vi "RT_Transmission.vi"() -> ()   [LabVIEW 2016]
uses:
  <vilib>/Instr/_visa.llb/VISA Configure Serial Port (Instr).vi
  <vilib>/FPGAPlugInAG/cRIO-9067/niLvFpga_Open_cRIO-9067.vi
  <vilib>/Utility/error.llb/Error Cluster From Error Code.vi
  <vilib>/rvi/errors/niLvFpgaAdjustHostInterfaceError.vi
  <vilib>/functionblocks/Control/PID/PID.vi
  <vilib>/rvi/interface/nirviOpenFPGA/nirviOpenFPGA.xnode
  FPGA Bitfiles/MayUpgrade_FPGA-Trans_Transmission-FPG_MZXtHOBdRVI.lvbitx
  FPGA_Transmission.vi
  <vilib>/rvi/interface/nirviReadWriteControl/nirviReadWriteControl.xnode
  <vilib>/functionblocks/FB Core/FB Core.xnode
  <vilib>/functionblocks/NI_FunctionBlock Libraries.lvlib
  NiFpgaLv.dll
  <vilib>/rvi/errors/niLvFpgaMergeErrorWithErrorCode.vi
panel:
  in  "Tab Control":enum32{"control", "Junk"}(tab)
  out "Steerer X+":dbl
  out "Steerer X-":dbl
  out "Steerer Y+":dbl
  out "Steerer Y-":dbl
  out "ExB +":dbl
  out "ExB -":dbl
  out "X+ V":fxp<+/-,26,5> format="%.23g"
  out "X+ I":fxp<+/-,26,5> format="%_4g"
  out "X- V":fxp<+/-,26,5> format="%_4g"
  out "X-I":fxp<+/-,26,5> format="%_4g"
  out "Y+ V":fxp<+/-,26,5> format="%_4g"
  out "Y+I":fxp<+/-,26,5> format="%_4g"
  out "Y-V":fxp<+/-,26,5> format="%_4g"
  out "Y-I":fxp<+/-,26,5> format="%_4g"
  out "ExB + V":fxp<+/-,26,5> format="%_4g"
  out "ExB +I":fxp<+/-,26,5> format="%_4g"
  out "ExB -V":fxp<+/-,26,5> format="%_4g"
  out "ExB-I":fxp<+/-,26,5> format="%_4g"
  out "concatenated string":string
  out "Ion gauge switch object cluser 2":T1
  out "Ion gauge anal waist Cluster 1":T1
  out "EXB":dbl
  in  "derivative time (Td, min)":dbl=0.05
  in  "integral time (Ti, min)":dbl=0.01
  in  "proportional gain (Kc)":dbl=25.0
  out "concatenated string 2":string
  out "anal field read":dbl
  out "unsigned byte array":u8[](array[numeric])
  out "Analyze read":u8[](array[numeric])
  out "analyze magnet set field":dbl
  out "element":dbl
  in  "diverter":bool
  out "diverter":bool
  out "ExB loop error":errorcluster
  out "Analog control error":errorcluster
  out "FPGA error":errorcluster
  in  "Ion gauge cluster control":T1
  out "Convectron 3":u8[](array[numeric])
  out "Ion gauge 4":u8[](array[numeric])
  out "Convectron 4":u8[](array[numeric])
  out "Ion gauge 5":u8[](array[numeric])
  out "Convectron 2":u8[](array[numeric])
  out "Ion gauge 2":u8[](array[numeric])
  out "Convectron 1":u8[](array[numeric])
  out "Ion gauge 1":u8[](array[numeric])
  out "Vac Cluster Error":errorcluster
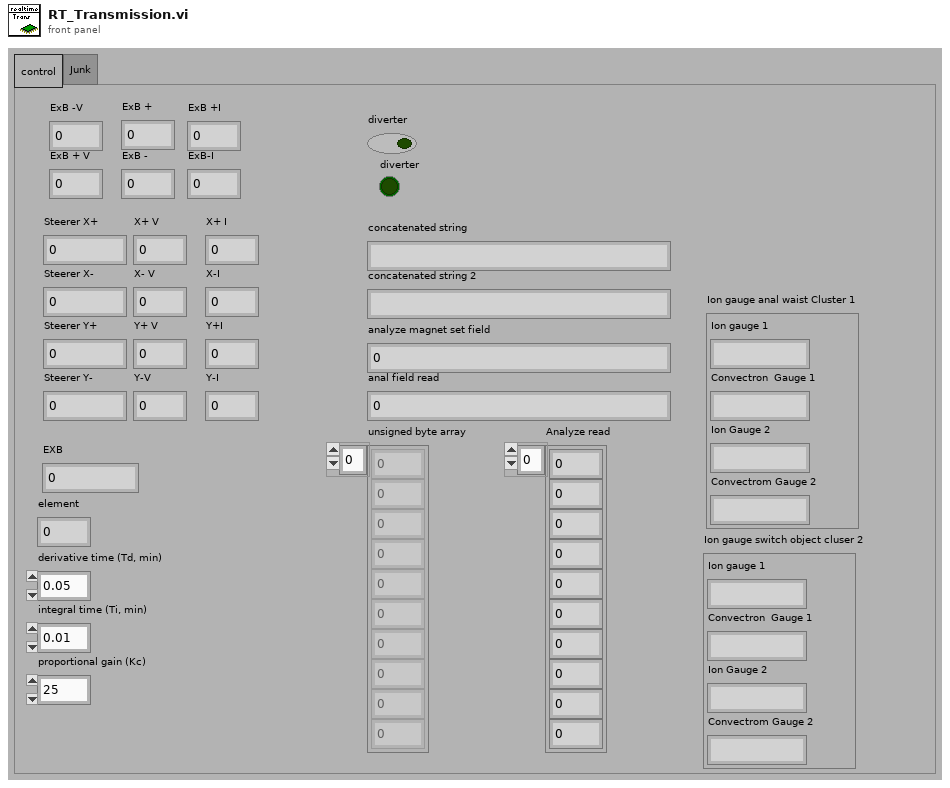
[diagram p1: front panel]
types:
  T1 = cluster{"Ion gauge 1":string, "Convectron  Gauge 1 ":string, "Ion Gauge 2":string, "Convectrom Gauge 2":string}
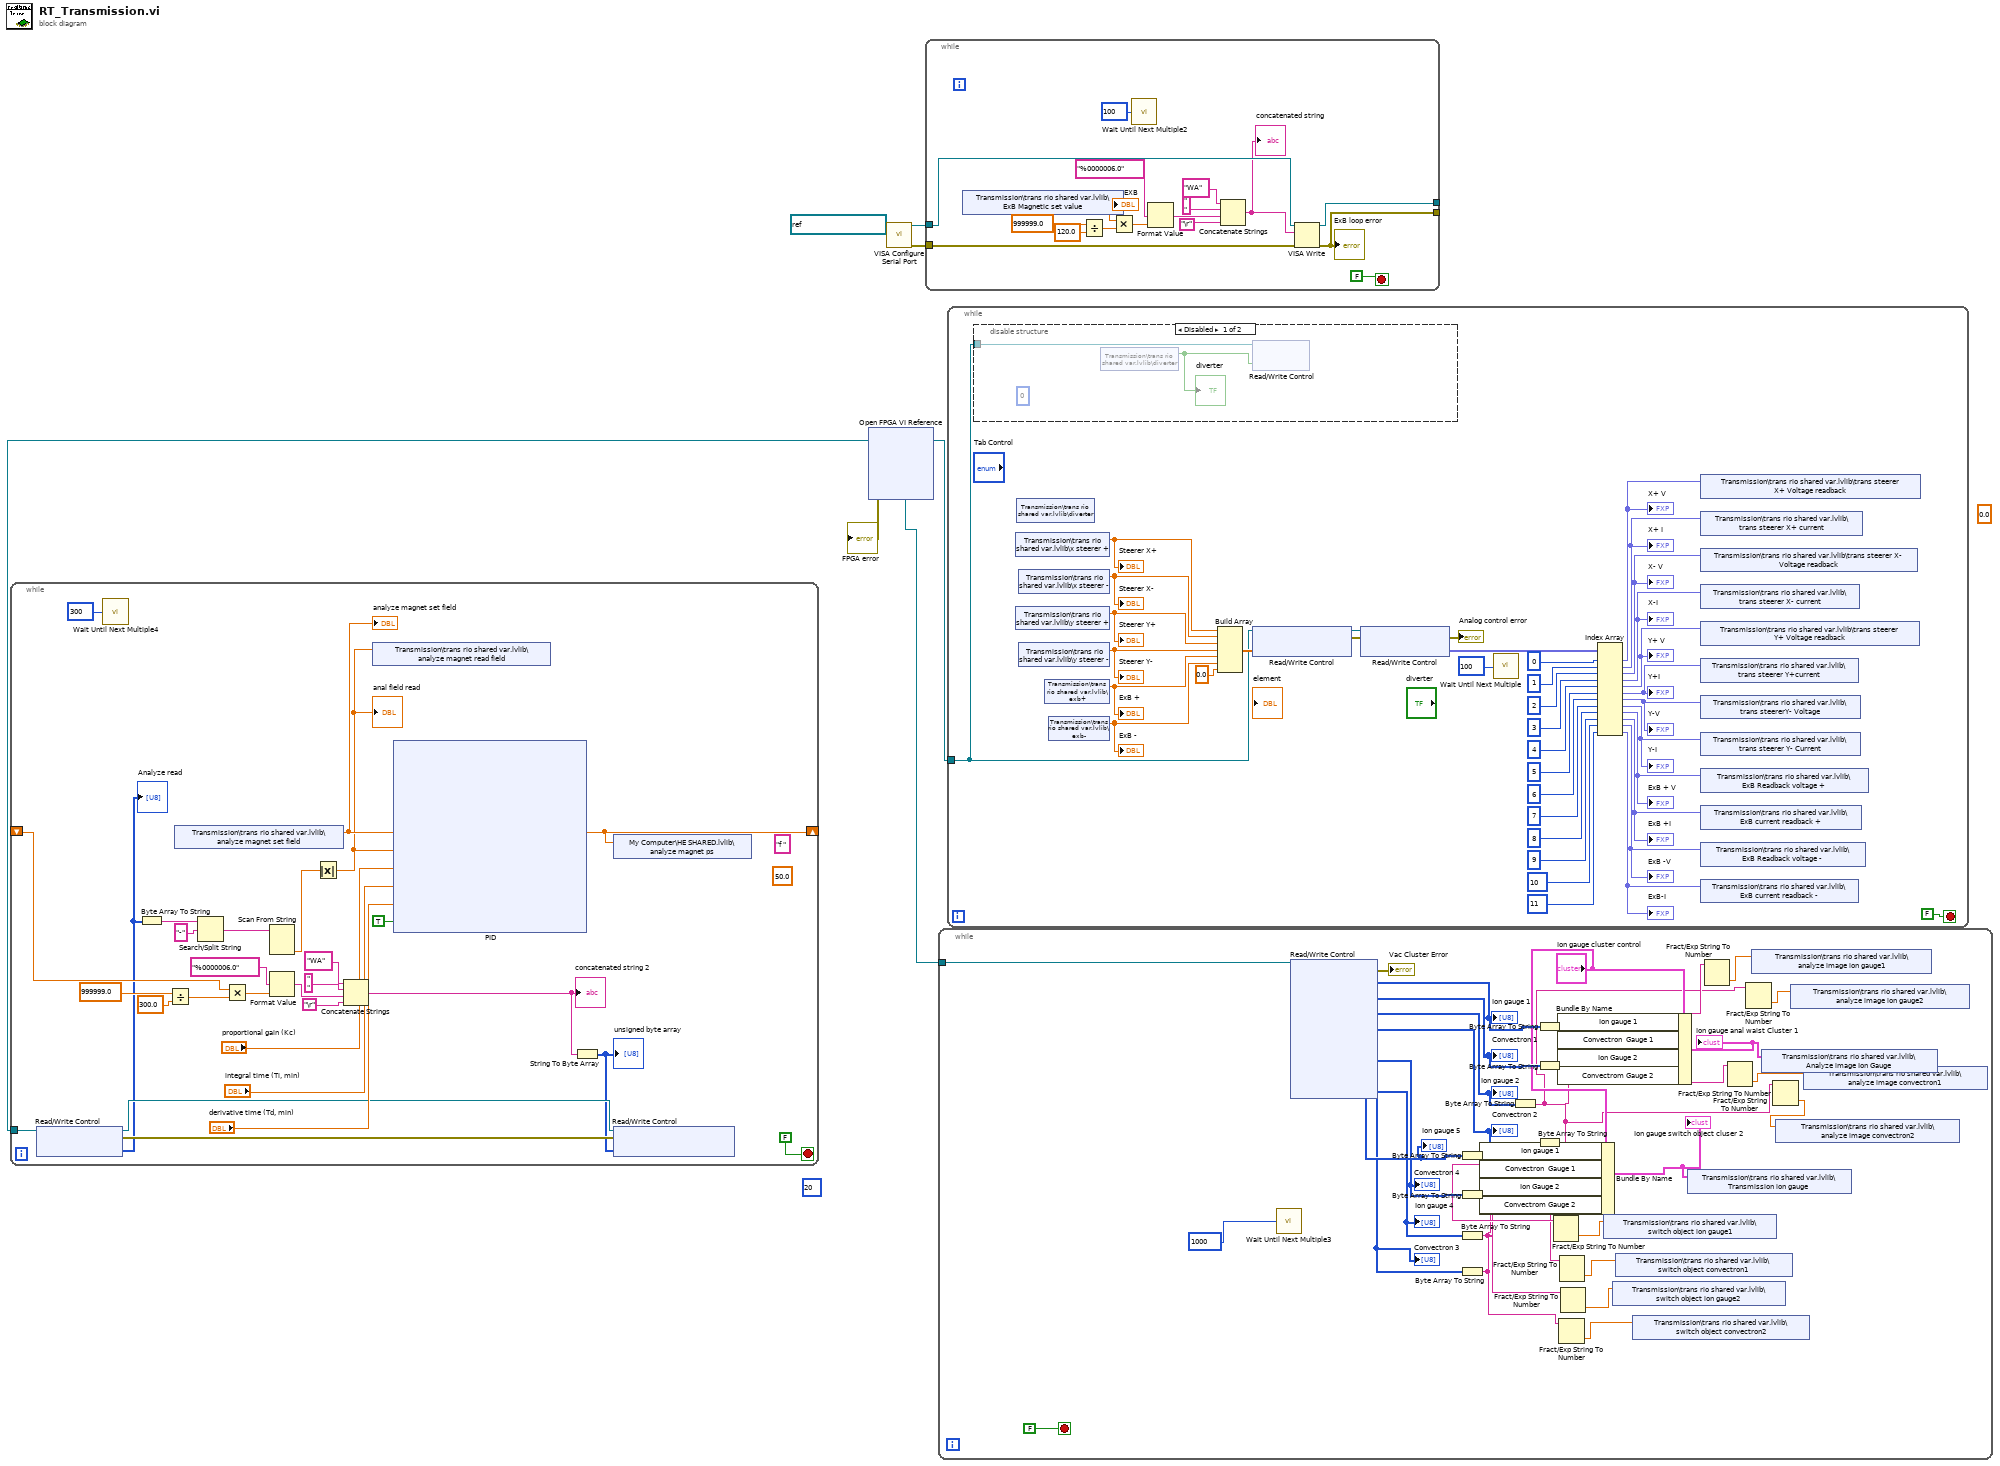
[diagram p0: block diagram]
diagram:
  (unwired) 20 ("dimension size")
  (unwired) 0.0 ("output")
  n1 = xnode "Open FPGA VI Reference"() -> ("FPGA VI Reference Out"=w1:refnum<k20>, "error out"=→"FPGA error":errorcluster)  [unwired: 2 in]
  n2 = while {
    shift-right: [w20] -> _
    shift-left: _ -> [w9]
    tunnel: w1 -> [w14]
    stop <- FALSE stop-if-true
    (unwired) 50.0 ("x")
    (unwired) "f " ("regular expression")
    n3 = xnode "Read/Write Control"("FPGA VI Reference In"=w14) -> ("FPGA VI Reference Out"=w13:refnum<k20>, "error out"=w12:errorcluster, "Analyze read"=w8:u8[])  [unwired: 1 in]
    "Analyze read" <- w8
    n4 = call "Wait Until Next Multiple4"("Count(mSec)"=u32 300 ("millisecond multiple")) -> ()  [unwired: 1 out]
    n5 = Byte Array To String(unsigned byte array=w8) -> (string=w22:string)
    n6 = Divide(x=999999.0, y=300.0) -> (x/y=w27:dbl)
    n7 = shared-variable "Transmission\\trans rio shared var.lvlib\\analyze magnet set field"() -> (w7:dbl)  [unwired: 1 in, 1 out]
    "analyze magnet set field" <- w7
    n8 = Search/Split String(string=w22, search string/char (-)="-") -> (match + rest of string=w10:string)  [unwired: 3 out]
    n9 = Multiply(x=w9, y=w27) -> (x*y=w29:dbl)
    n10 = Scan From String(input string=w10) -> (output 1=w21:dbl)  [unwired: 3 in, 4 out]
    n11 = Format Value(format string="%0000006.0", value (0)=w29) -> (output string=w32:string)  [unwired: 1 out]
    n12 = Absolute Value(x=w21) -> (abs(x)=w6:dbl)
    "anal field read" <- w6
    n13 = Concatenate Strings("WA", " ", w32, "\r") -> (w33:string)
    "concatenated string 2" <- w33
    n14 = shared-variable "Transmission\\trans rio shared var.lvlib\\analyze magnet read field"(w6) -> ()  [unwired: 1 in, 1 out]
    n15 = xnode "PID"("setpoint"=w7, "process variable"=w6, "proportional gain (Kc)"="proportional gain (Kc)", "integral time (Ti, min)"="integral time (Ti, min)", "derivative time (Td, min)"="derivative time (Td, min)", "auto? (T)"=TRUE) -> ("output"=w20:dbl)  [unwired: 1 in, 1 out]
    n16 = String To Byte Array(string=w33) -> (unsigned byte array=w11:u8[])
    "unsigned byte array" <- w11
    n17 = shared-variable "My Computer\\HE SHARED.lvlib\\analyze magnet ps"(w20) -> ()  [unwired: 1 in, 1 out]
    n18 = xnode "Read/Write Control"("FPGA VI Reference In"=w13, "error in"=w12, "analyze ps set array"=w11) -> ()  [unwired: 2 out]
  }
  n19 = call-poly "VISA Configure Serial Port"("VISA resource name"=refnum<visa-resource-name> "ASRL1::INSTR") -> ("VISA resource name out"=w5:refnum<visa-resource-name>, "error out"=w4:errorcluster)  [unwired: 5 in, 8 out]
  n20 = while {
    tunnel: w4 -> [w107]
    tunnel: w5 -> [w106]
    tunnel: [w104] -> _
    tunnel: [w103] -> _
    stop <- FALSE stop-if-true
    n21 = shared-variable "Transmission\\trans rio shared var.lvlib\\ExB Magnetic set value"() -> (w102:dbl)  [unwired: 1 in, 1 out]
    "EXB" <- w102
    n22 = Divide(x=999999.0, y=120.0) -> (x/y=w115:dbl)
    n23 = Multiply(x=w102, y=w115) -> (x*y=w108:dbl)
    n24 = call "Wait Until Next Multiple2"("Count(mSec)"=u32 100) -> ()  [unwired: 1 out]
    n25 = Format Value(format string="%0000006.0", value (0)=w108) -> (output string=w111:string)  [unwired: 1 out]
    n26 = Concatenate Strings("WA", " ", w111, "\r") -> (w105:string)
    "concatenated string" <- w105
    n27 = VISA Write(VISA resource name=w106, write buffer=w105, error in (no error)=w107) -> (VISA resource name out=w104:refnum<visa-resource-name>, error out=w103:errorcluster)  [unwired: 1 out]
    "ExB loop error" <- w103
  }
  n28 = while {
    tunnel: w1 -> [w136]
    stop <- FALSE stop-if-true
    n29 = call "Wait Until Next Multiple3"("Count(mSec)"=u32 1000 ("millisecond multiple")) -> ()  [unwired: 1 out]
    n30 = xnode "Read/Write Control"("FPGA VI Reference In"=w136) -> ("error out"=→"Vac Cluster Error":errorcluster, "Ion gauge 1"=w145:u8[], "Convectron 1"=w146:u8[], "Ion gauge 2"=w147:u8[], "Convectron 2"=w148:u8[], "Ion gauge 3"=w142:u8[], "Convectron 3"=w141:u8[], "Convectron 4"=w139:u8[], "Ion gauge 4"=w140:u8[])  [unwired: 1 in, 1 out]
    "Ion gauge 1" <- w145
    "Convectron 1" <- w146
    "Ion gauge 2" <- w147
    "Convectron 2" <- w148
    "Ion gauge 5" <- w142
    "Convectron 4" <- w141
    "Ion gauge 4" <- w140
    "Convectron 3" <- w139
    n31 = Byte Array To String(unsigned byte array=w142) -> (string=w133:string)
    n32 = Byte Array To String(unsigned byte array=w141) -> (string=w132:string)
    n33 = Byte Array To String(unsigned byte array=w140) -> (string=w131:string)
    n34 = Byte Array To String(unsigned byte array=w139) -> (string=w130:string)
    n35 = Bundle By Name(cluster="Ion gauge cluster control", "Ion gauge 1"=w133, "Convectron  Gauge 1"=w132, "Ion Gauge 2"=w131, "Convectrom Gauge 2"=w130) -> (w135:T1)
    "Ion gauge switch object cluser 2" <- w135
    n36 = Byte Array To String(unsigned byte array=w147) -> (string=w122:string)
    n37 = Byte Array To String(unsigned byte array=w145) -> (string=w125:string)
    n38 = Byte Array To String(unsigned byte array=w146) -> (string=w124:string)
    n39 = Byte Array To String(unsigned byte array=w148) -> (string=w123:string)
    n40 = Fract/Exp String To Number(string=w133) -> (number=w129:dbl)  [unwired: 3 in, 1 out]
    n41 = Bundle By Name(cluster="Ion gauge cluster control", "Ion gauge 1"=w125, "Convectron  Gauge 1"=w124, "Ion Gauge 2"=w122, "Convectrom Gauge 2"=w123) -> (w134:T1)
    "Ion gauge anal waist Cluster 1" <- w134
    n42 = Fract/Exp String To Number(string=w130) -> (number=w126:dbl)  [unwired: 3 in, 1 out]
    n43 = Fract/Exp String To Number(string=w132) -> (number=w128:dbl)  [unwired: 3 in, 1 out]
    n44 = Fract/Exp String To Number(string=w131) -> (number=w127:dbl)  [unwired: 3 in, 1 out]
    n45 = shared-variable "Transmission\\trans rio shared var.lvlib\\switch object ion gauge1"(w129) -> ()  [unwired: 1 in, 1 out]
    n46 = shared-variable "Transmission\\trans rio shared var.lvlib\\switch object ion gauge2"(w127) -> ()  [unwired: 1 in, 1 out]
    n47 = shared-variable "Transmission\\trans rio shared var.lvlib\\switch object convectron1"(w128) -> ()  [unwired: 1 in, 1 out]
    n48 = shared-variable "Transmission\\trans rio shared var.lvlib\\switch object convectron2"(w126) -> ()  [unwired: 1 in, 1 out]
    n49 = shared-variable "Transmission\\trans rio shared var.lvlib\\Transmission ion gauge"(w135) -> ()  [unwired: 1 in, 1 out]
    n50 = Fract/Exp String To Number(string=w125) -> (number=w121:dbl)  [unwired: 3 in, 1 out]
    n51 = Fract/Exp String To Number(string=w124) -> (number=w119:dbl)  [unwired: 3 in, 1 out]
    n52 = Fract/Exp String To Number(string=w122) -> (number=w120:dbl)  [unwired: 3 in, 1 out]
    n53 = shared-variable "Transmission\\trans rio shared var.lvlib\\analyze image ion gauge1"(w121) -> ()  [unwired: 1 in, 1 out]
    n54 = shared-variable "Transmission\\trans rio shared var.lvlib\\Analyze image Ion Gauge"(w134) -> ()  [unwired: 1 in, 1 out]
    n55 = Fract/Exp String To Number(string=w123) -> (number=w118:dbl)  [unwired: 3 in, 1 out]
    n56 = shared-variable "Transmission\\trans rio shared var.lvlib\\analyze image convectron2"(w118) -> ()  [unwired: 1 in, 1 out]
    n57 = shared-variable "Transmission\\trans rio shared var.lvlib\\analyze image ion gauge2"(w120) -> ()  [unwired: 1 in, 1 out]
    n58 = shared-variable "Transmission\\trans rio shared var.lvlib\\analyze image convectron1"(w119) -> ()  [unwired: 1 in, 1 out]
  }
  n59 = while {
    tunnel: w1 -> [w149]
    stop <- FALSE stop-if-true
    n60 = disable-structure shown="Disabled" {
      disable-tunnel: w149 -> [w189 _]
      frame Disabled {
        (unwired) 0 ("dimension size")
        n61 = shared-variable "Transmission\\trans rio shared var.lvlib\\diverter"() -> (w188:bool)  [unwired: 1 in, 1 out]
        "diverter" <- w188
        n62 = xnode "Read/Write Control"("FPGA VI Reference In"=w189, "diverter"=w188) -> ()  [unwired: 1 in, 2 out]
      }
      frame Enabled {
      }
    }
    n63 = shared-variable "Transmission\\trans rio shared var.lvlib\\x steerer +"() -> (w168:dbl)  [unwired: 1 in, 1 out]
    "Steerer X+" <- w168
    n64 = shared-variable "Transmission\\trans rio shared var.lvlib\\y steerer +"() -> (w170:dbl)  [unwired: 1 in, 1 out]
    "Steerer Y+" <- w170
    n65 = shared-variable "Transmission\\trans rio shared var.lvlib\\diverter"() -> ()  [unwired: 1 in, 2 out]
    n66 = shared-variable "Transmission\\trans rio shared var.lvlib\\x steerer -"() -> (w169:dbl)  [unwired: 1 in, 1 out]
    "Steerer X-" <- w169
    n67 = shared-variable "Transmission\\trans rio shared var.lvlib\\y steerer -"() -> (w171:dbl)  [unwired: 1 in, 1 out]
    "Steerer Y-" <- w171
    n68 = shared-variable "Transmission\\trans rio shared var.lvlib\\exb+"() -> (w172:dbl)  [unwired: 1 in, 1 out]
    "ExB +" <- w172
    n69 = shared-variable "Transmission\\trans rio shared var.lvlib\\exb-"() -> (w173:dbl)  [unwired: 1 in, 1 out]
    "ExB -" <- w173
    n70 = Build Array(w168, w169, w170, w171, w172, w173, 0.0 ("element")) -> (w187:dbl[])
    n71 = xnode "Read/Write Control"("FPGA VI Reference In"=w149, "Analog Output"=w187) -> ("FPGA VI Reference Out"=w153:refnum<k20>, "error out"=w152:errorcluster)  [unwired: 1 in]
    n72 = xnode "Read/Write Control"("FPGA VI Reference In"=w153, "error in"=w152) -> ("error out"=→"Analog control error":errorcluster, "Analog input"=w154:fxp<+/-,26,5>[])  [unwired: 1 out]
    n73 = call "Wait Until Next Multiple"("Count(mSec)"=u32 100) -> ()  [unwired: 1 out]
    n74 = Index Array(array=w154, index #1=0 ("index"), index #2=1 ("index"), index #3=2 ("index"), index #4=3 ("index"), index #5=4 ("index"), index #6=5 ("index"), index #7=6 ("index"), index #8=7 ("index"), index #9=8 ("index"), index #10=9 ("index"), index #11=10 ("index"), index #12=11 ("index")) -> (element #1=w166:fxp<+/-,26,5>, element #2=w164:fxp<+/-,26,5>, element #3=w165:fxp<+/-,26,5>, element #4=w167:fxp<+/-,26,5>, element #5=w163:fxp<+/-,26,5>, element #6=w161:fxp<+/-,26,5>, element #7=w162:fxp<+/-,26,5>, element #8=w160:fxp<+/-,26,5>, element #9=w159:fxp<+/-,26,5>, element #10=w157:fxp<+/-,26,5>, element #11=w158:fxp<+/-,26,5>, element #12=w156:fxp<+/-,26,5>)
    "X+ V" <- w166
    "X+ I" <- w164
    "X- V" <- w165
    "X-I" <- w167
    "Y+ V" <- w163
    "Y+I" <- w161
    "Y-V" <- w162
    "Y-I" <- w160
    "ExB + V" <- w159
    "ExB +I" <- w157
    "ExB -V" <- w158
    "ExB-I" <- w156
    n75 = shared-variable "Transmission\\trans rio shared var.lvlib\\trans steerer X+ Voltage readback"(w166) -> ()  [unwired: 1 in, 1 out]
    n76 = shared-variable "Transmission\\trans rio shared var.lvlib\\trans steerer X+ current"(w164) -> ()  [unwired: 1 in, 1 out]
    n77 = shared-variable "Transmission\\trans rio shared var.lvlib\\trans steerer X- Voltage readback"(w165) -> ()  [unwired: 1 in, 1 out]
    n78 = shared-variable "Transmission\\trans rio shared var.lvlib\\trans steerer X- current"(w167) -> ()  [unwired: 1 in, 1 out]
    n79 = shared-variable "Transmission\\trans rio shared var.lvlib\\trans steerer Y+ Voltage readback"(w163) -> ()  [unwired: 1 in, 1 out]
    n80 = shared-variable "Transmission\\trans rio shared var.lvlib\\trans steerer Y+current"(w161) -> ()  [unwired: 1 in, 1 out]
    n81 = shared-variable "Transmission\\trans rio shared var.lvlib\\trans steererY- Voltage"(w162) -> ()  [unwired: 1 in, 1 out]
    n82 = shared-variable "Transmission\\trans rio shared var.lvlib\\trans steerer Y- Current"(w160) -> ()  [unwired: 1 in, 1 out]
    n83 = shared-variable "Transmission\\trans rio shared var.lvlib\\ExB Readback voltage +"(w159) -> ()  [unwired: 1 in, 1 out]
    n84 = shared-variable "Transmission\\trans rio shared var.lvlib\\ExB current readback +"(w157) -> ()  [unwired: 1 in, 1 out]
    n85 = shared-variable "Transmission\\trans rio shared var.lvlib\\ExB Readback voltage -"(w158) -> ()  [unwired: 1 in, 1 out]
    n86 = shared-variable "Transmission\\trans rio shared var.lvlib\\ExB current readback -"(w156) -> ()  [unwired: 1 in, 1 out]
  }
